vi "SVN_Info.vi"(5 "rev End":i32=-2, 8 "Error In":errorcluster, 11 "repo path":path=path "") -> (0 "Error Out":errorcluster, 3 "SVN_Info_Cluster":T1)   [LabVIEW 2014]
uses:
  controls/SVN_LogEntry_Cluster.ctl
  controls/SVN_Info_Cluster.ctl
panel:
  out "cmd command":string
  out "standard output":string
  out "standard error":string
  # "This VI queries a single SVN log entry"
  # "DATE -1\nHEAD -2\nBASE -3\nCOMMITED -4\nPREV -5"
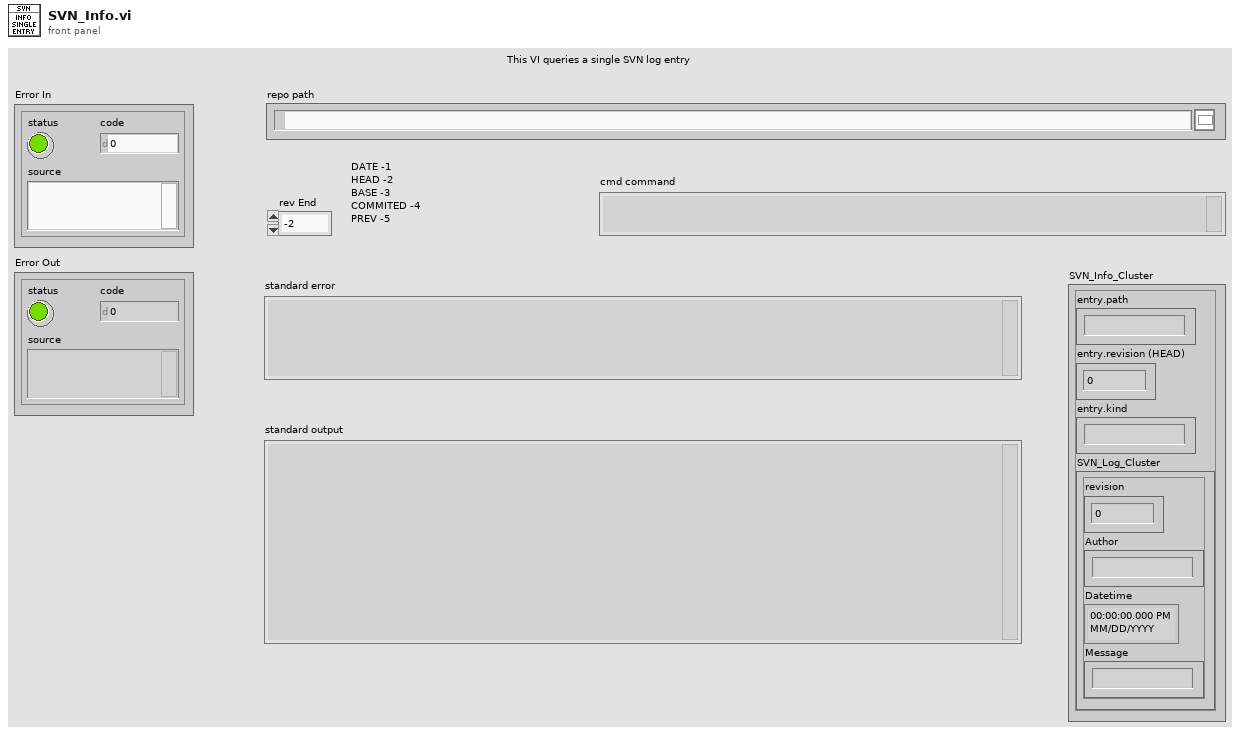
[diagram p1: front panel]
types:
  T1 = typedef "SVN_Info_Cluster.ctl" = cluster{"entry.path":string, "entry.revision (HEAD)":i32, "entry.kind":string, "SVN_Log_Cluster":T2}
  T2 = typedef "SVN_LogEntry_Cluster.ctl" = cluster{"revision":i32, "Author":string, "Datetime":timestamp, "Message":string}
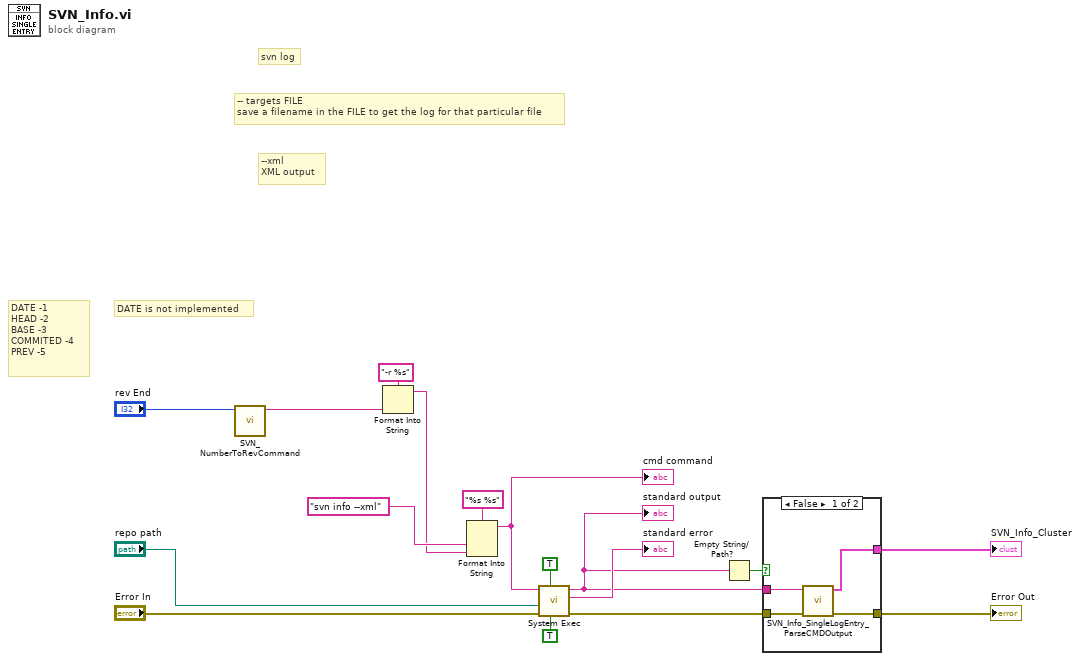
[diagram p0: block diagram]
diagram:
  # "DATE is not implemented"
  # "DATE -1\nHEAD -2\nBASE -3\nCOMMITED -4\nPREV -5"
  # "--xml\nXML output"
  # "-- targets FILE \nsave a filename in the FILE to get the log for that particular file"
  # "svn log"
  n1 = call "SVN_NumberToRevCommand.vi"("rev End"="rev End") -> ("String"=w10:string)  [unwired: 10 in]
  n2 = Format Into String(format string="-r %s", w10) -> (resulting string=w7:string)  [unwired: 2 in, 1 out]
  n3 = Format Into String(format string="%s %s", "svn info --xml" ("command line"), w7) -> (resulting string=w5:string)  [unwired: 2 in, 1 out]
  "cmd command" <- w5
  n4 = call <vilib>:"System Exec.vi"("run minimized? (F)"=TRUE, "wait until completion? (T)"=TRUE, "error in (no error)"="Error In", "working directory"="repo path", "command line"=w5) -> ("error out"=w3:errorcluster, "standard error"=→"standard error":string, "standard output"=w6:string)  [unwired: 3 in, 1 out]
  "standard output" <- w6
  n5 = Empty String/Path?(string/path=w6) -> (empty?=w4:bool)
  n6 = case shown="False" w4 {
    tunnel: w6 -> [w19 _]
    tunnel: w3 -> [w20 w22]
    tunnel: [w21 w22] -> w2
    tunnel: [w18 _] -> w1
    frame False {
      n7 = call "SVN_Info_SingleLogEntry_ParseCMDOutput.vi"("Error In"=w20, "SVN_Log_XML (In)"=w19) -> ("Error Out"=w21:errorcluster, "SVN_Info_Cluster"=w18:T1)  [unwired: 8 in]
    }
    frame True {
    }
  }
  "Error Out" <- w2
  "SVN_Info_Cluster" <- w1
